vi "输入数据解析.vi"(0 "单个参数补充":dbl, 1 "从板号":dbl=1.0, 2 "主板二维码":string="BNET01", 3 "从板二维码":string="BNET01", 5 "主板引用":refnum<vi>, 7 "从板引用":refnum<vi>, 9 "主板选项":string="三级故障阀值", 11 "枚举":enum16{"主板", "从板"}(ring), 12 "快换":bool caption="快换写入") -> (4 "输出数组":dbl[][](array[numeric]), 6 "数组长度":dbl[](array[numeric]), 8 "循环次数":i32, 10 "命令":u32, 14 "名称":string[](array[string]), 15 "命令序号":u32[](array[numeric]))   [LabVIEW 2013] (continued)
                n2255 = Unbundle By Name(w5791) -> ("SOC过低"=w5790:dbl)
                n2256 = call "输入分辨率计算-EV05.vi"("1字节?"=FALSE, "数值"=w5790, "偏移量"=0.0, "分辨率"=0.1) -> ("低字节"=w5788:dbl, "高字节1"=w5789:dbl)  [unwired: 1 in, 5 out]
                n2257 = call "二进制解析-8.6.vi"("索引"=4, "数值"=w5789) -> ("低位子数组"=w5787:i32[])  [unwired: 3 out]
                n2258 = disable-structure shown="启用" {
                  disable-tunnel: w5788 -> [w5798 _]
                  disable-tunnel: [w5798 255 ("高字节1")] -> w5786
                  disable-tunnel: w5787 -> [w5797 _]
                  frame Disabled {
                    (unwired) i32[] [] ("低位子数组 4")
                  }
                  frame Enabled {
                  }
                }
                n2259 = Build Array(w5786, w5786) -> (w5794:i32[])
              }
              frame 14 {
                # "内阻过大"
                n2260 = disable-structure shown="启用" {
                  disable-tunnel: w5802 -> [w5807 _]
                  disable-tunnel: [w5803 255 ("高字节1")] -> w5800
                  frame Disabled {
                    n2261 = Unbundle By Name(w5807) -> ("内阻过大"=w5806:dbl)
                    n2262 = call "输入分辨率计算-EV05.vi"("1字节?"=TRUE, "数值"=w5806, "分辨率"=0.1) -> ("高字节1"=w5803:dbl)  [unwired: 2 in, 6 out]
                  }
                  frame Enabled {
                  }
                }
                n2263 = Build Array(w5800) -> (w5801:i32[])
              }
              frame 15 {
                # "极柱温度过高"
                n2264 = disable-structure shown="启用" {
                  disable-tunnel: w5811 -> [w5817 _]
                  disable-tunnel: [w5813 255 ("高字节1")] -> w5809
                  frame Disabled {
                    n2265 = Unbundle By Name(w5817) -> ("极柱温度过高"=w5816:dbl)
                    n2266 = call "输入分辨率计算-EV05.vi"("1字节?"=TRUE, "数值"=w5816, "偏移量"=-40.0, "分辨率"=1.0) -> ("高字节1"=w5813:dbl)  [unwired: 1 in, 6 out]
                  }
                  frame Enabled {
                  }
                }
                n2267 = Build Array(w5809) -> (w5810:i32[])
              }
              frame 16 {
                # "SOH过低"
                n2268 = disable-structure shown="启用" {
                  disable-tunnel: [w5834 w5842] -> w5821
                  disable-tunnel: w5820 -> [w5831 _]
                  disable-tunnel: [w5823 w5842] -> w5819
                  frame Disabled {
                    n2269 = Unbundle By Name(w5831) -> ("SOH过低"=w5830:dbl)
                    n2270 = call "输入分辨率计算-EV05.vi"("1字节?"=FALSE, "数值"=w5830, "偏移量"=0.0, "分辨率"=0.1) -> ("低字节"=w5832:dbl, "高字节1"=w5833:dbl)  [unwired: 1 in, 5 out]
                    n2271 = call "二进制解析-8.6.vi"("索引"=4, "数值"=w5833) -> ("低位子数组"=w5836:i32[])  [unwired: 3 out]
                    n2272 = call "二进制解析-8.6.vi"("索引"=4, "数值"=w5832) -> ("低位子数组"=w5825:i32[], "高位子数组"=w5835:i32[])  [unwired: 2 out]
                    n2273 = call "二进制解析-8.6.vi"("索引"=4, "数值"=0) -> ("低位子数组"=w5826:i32[])  [unwired: 3 out]
                    n2274 = Insert Into Array(array=w5836, new element=w5835) -> (w5829:i32[])  [unwired: 1 in]
                    n2275 = Insert Into Array(array=w5825, new element=w5826) -> (w5824:i32[])  [unwired: 1 in]
                    n2276 = call "数值二进制转十进制-8.6.vi"("子数组"=w5829) -> ("十进制数值"=w5834:i32)  [unwired: 4 out]
                    n2277 = call "数值二进制转十进制-8.6.vi"("子数组"=w5824) -> ("十进制数值"=w5823:i32)  [unwired: 4 out]
                  }
                  frame Enabled {
                    w5842 = 255 ("高字节1")
                  }
                }
                n2278 = Build Array(w5821, w5819) -> (w5822:i32[])
              }
            }
            n2279 = Insert Into Array(array=w5628, new element=w5629) -> (w5627:dbl[])  [unwired: 1 in]
          }
          n2280 = Build Array(w5624) -> (w5623:dbl[][])
          n2281 = Build Array("三级故障阀值") -> (w5614:string[])
        }
        frame "单体电压过高" {
          n2282 = Unbundle By Name(w5848) -> ("一级故障"=w5849:refnum<vi>)
          n2283 = property class="Clust (严格)"(reference=w5849) -> ("Value"=w5847:T4)  [unwired: 1 in, 2 out]
          n2284 = for {
            N: 17 -> [_]
            tunnel: w5847 -> [w5859]
            shift-right: [w5856] -> w5853
            shift-left: dbl[] [] -> [w5857]
            i -> [w5860]
            n2285 = case shown="13" w5860 {
              tunnel: w5859 -> [w5861 w5872 w5883 w5893 w5903 w5913 w5925 w5937 w5949 w5961 w5973 w5985 w5999 w6020 w6032 w6041 w6050]
              tunnel: [w5862 w5873 w5884 w5894 w5904 w5915 w5927 w5939 w5951 w5963 w5975 w5986 w6008 w6023 w6031 w6040 w6052] -> w5858
              frame 0, Default {
                # "总电压过高"
                n2286 = disable-structure shown="启用" {
                  disable-tunnel: [w5868 w5871] -> w5864
                  disable-tunnel: [w5867 w5871] -> w5863
                  disable-tunnel: w5861 -> [w5866 _]
                  frame Disabled {
                    n2287 = Unbundle By Name(w5866) -> ("总电压过高"=w5865:dbl)
                    n2288 = call "输入分辨率计算-EV05.vi"("1字节?"=FALSE, "数值"=w5865, "分辨率"=0.1) -> ("低字节"=w5868:dbl, "高字节1"=w5867:dbl)  [unwired: 2 in, 5 out]
                  }
                  frame Enabled {
                    w5871 = 255 ("高字节1")
                  }
                }
                n2289 = Build Array(w5863, w5864) -> (w5862:i32[])
              }
              frame 1 {
                # "总电压过低"
                n2290 = disable-structure shown="启用" {
                  disable-tunnel: [w5879 w5882] -> w5875
                  disable-tunnel: [w5878 w5882] -> w5874
                  disable-tunnel: w5872 -> [w5877 _]
                  frame Disabled {
                    n2291 = Unbundle By Name(w5877) -> ("总电压过低"=w5876:dbl)
                    n2292 = call "输入分辨率计算-EV05.vi"("1字节?"=FALSE, "数值"=w5876, "分辨率"=0.1) -> ("低字节"=w5879:dbl, "高字节1"=w5878:dbl)  [unwired: 2 in, 5 out]
                  }
                  frame Enabled {
                    w5882 = 255 ("高字节1")
                  }
                }
                n2293 = Build Array(w5874, w5875) -> (w5873:i32[])
              }
              frame 2 {
                # "温度过高"
                n2294 = disable-structure shown="启用" {
                  disable-tunnel: [w5889 255 ("高字节1")] -> w5885
                  disable-tunnel: w5883 -> [w5887 _]
                  frame Disabled {
                    n2295 = Unbundle By Name(w5887) -> ("温度过高"=w5886:dbl)
                    n2296 = call "输入分辨率计算-EV05.vi"("1字节?"=TRUE, "数值"=w5886, "偏移量"=-40.0, "分辨率"=1.0) -> ("高字节1"=w5889:dbl)  [unwired: 1 in, 6 out]
                  }
                  frame Enabled {
                  }
                }
                n2297 = Build Array(w5885) -> (w5884:i32[])
              }
              frame 3 {
                # "温度过低"
                n2298 = disable-structure shown="启用" {
                  disable-tunnel: [w5899 255 ("高字节1")] -> w5895
                  disable-tunnel: w5893 -> [w5897 _]
                  frame Disabled {
                    n2299 = Unbundle By Name(w5897) -> ("温度过低"=w5896:dbl)
                    n2300 = call "输入分辨率计算-EV05.vi"("1字节?"=TRUE, "数值"=w5896, "偏移量"=-40.0, "分辨率"=1.0) -> ("高字节1"=w5899:dbl)  [unwired: 1 in, 6 out]
                  }
                  frame Enabled {
                  }
                }
                n2301 = Build Array(w5895) -> (w5894:i32[])
              }
              frame 4 {
                # "整组温度不均衡"
                n2302 = disable-structure shown="启用" {
                  disable-tunnel: [w5909 255 ("高字节1")] -> w5905
                  disable-tunnel: w5903 -> [w5907 _]
                  frame Disabled {
                    n2303 = Unbundle By Name(w5907) -> ("整组温度不均衡"=w5906:dbl)
                    n2304 = call "输入分辨率计算-EV05.vi"("1字节?"=TRUE, "数值"=w5906, "偏移量"=0.0, "分辨率"=1.0) -> ("高字节1"=w5909:dbl)  [unwired: 1 in, 6 out]
                  }
                  frame Enabled {
                  }
                }
                n2305 = Build Array(w5905) -> (w5904:i32[])
              }
              frame 5 {
                # "单组电压不均衡"
                n2306 = disable-structure shown="启用" {
                  disable-tunnel: [w5921 w5924] -> w5916
                  disable-tunnel: [w5919 w5924] -> w5914
                  disable-tunnel: w5913 -> [w5918 _]
                  frame Disabled {
                    n2307 = Unbundle By Name(w5918) -> ("单组电压不均衡"=w5917:dbl)
                    n2308 = call "输入分辨率计算-EV05.vi"("1字节?"=FALSE, "数值"=w5917, "偏移量"=0.0, "分辨率"=0.001) -> ("低字节"=w5919:dbl, "高字节1"=w5921:dbl)  [unwired: 1 in, 5 out]
                  }
                  frame Enabled {
                    w5924 = 255 ("高字节1")
                  }
                }
                n2309 = Build Array(w5916, w5914) -> (w5915:i32[])
              }
              frame 6 {
                # "整组电压不均衡"
                n2310 = disable-structure shown="启用" {
                  disable-tunnel: [w5933 w5936] -> w5928
                  disable-tunnel: [w5931 w5936] -> w5926
                  disable-tunnel: w5925 -> [w5930 _]
                  frame Disabled {
                    n2311 = Unbundle By Name(w5930) -> ("整组电压不均衡"=w5929:dbl)
                    n2312 = call "输入分辨率计算-EV05.vi"("1字节?"=FALSE, "数值"=w5929, "偏移量"=0.0, "分辨率"=0.001) -> ("低字节"=w5931:dbl, "高字节1"=w5933:dbl)  [unwired: 1 in, 5 out]
                  }
                  frame Enabled {
                    w5936 = 255 ("高字节1")
                  }
                }
                n2313 = Build Array(w5928, w5926) -> (w5927:i32[])
              }
              frame 7 {
                # "单体电压过高"
                n2314 = disable-structure shown="启用" {
                  disable-tunnel: [w5945 w5948] -> w5940
                  disable-tunnel: [w5943 w5948] -> w5938
                  disable-tunnel: w5937 -> [w5942 _]
                  frame Enabled {
                    n2315 = Unbundle By Name(w5942) -> ("单体电压过高"=w5941:dbl)
                    n2316 = call "输入分辨率计算-EV05.vi"("1字节?"=FALSE, "数值"=w5941, "偏移量"=0.0, "分辨率"=0.001) -> ("低字节"=w5943:dbl, "高字节1"=w5945:dbl)  [unwired: 1 in, 5 out]
                  }
                  frame Disabled {
                    w5948 = 255 ("高字节1")
                  }
                }
                n2317 = Build Array(w5940, w5938) -> (w5939:dbl[])
              }
              frame 8 {
                # "单体电压过低"
                n2318 = disable-structure shown="启用" {
                  disable-tunnel: [w5957 w5960] -> w5952
                  disable-tunnel: [w5955 w5960] -> w5950
                  disable-tunnel: w5949 -> [w5954 _]
                  frame Disabled {
                    n2319 = Unbundle By Name(w5954) -> ("单体电压过低"=w5953:dbl)
                    n2320 = call "输入分辨率计算-EV05.vi"("1字节?"=FALSE, "数值"=w5953, "偏移量"=0.0, "分辨率"=0.001) -> ("低字节"=w5955:dbl, "高字节1"=w5957:dbl)  [unwired: 1 in, 5 out]
                  }
                  frame Enabled {
                    w5960 = 255 ("高字节1")
                  }
                }
                n2321 = Build Array(w5952, w5950) -> (w5951:i32[])
              }
              frame 9 {
                # "充电电流过高"
                n2322 = disable-structure shown="启用" {
                  disable-tunnel: [w5969 w5972] -> w5964
                  disable-tunnel: [w5967 w5972] -> w5962
                  disable-tunnel: w5961 -> [w5966 _]
                  frame Disabled {
                    n2323 = Unbundle By Name(w5966) -> ("充电电流过高"=w5965:dbl)
                    n2324 = call "输入分辨率计算-EV05.vi"("1字节?"=FALSE, "数值"=w5965, "偏移量"=-3000.0, "分辨率"=0.1) -> ("低字节"=w5967:dbl, "高字节1"=w5969:dbl)  [unwired: 1 in, 5 out]
                  }
                  frame Enabled {
                    w5972 = 255 ("高字节1")
                  }
                }
                n2325 = Build Array(w5964, w5962) -> (w5963:i32[])
              }
              frame 10 {
                # "放电电流过高"
                n2326 = disable-structure shown="启用" {
                  disable-tunnel: [w5981 w5984] -> w5976
                  disable-tunnel: [w5979 w5984] -> w5974
                  disable-tunnel: w5973 -> [w5978 _]
                  frame Disabled {
                    n2327 = Unbundle By Name(w5978) -> ("放电电流过高"=w5977:dbl)
                    n2328 = call "输入分辨率计算-EV05.vi"("1字节?"=FALSE, "数值"=w5977, "偏移量"=-3000.0, "分辨率"=0.1) -> ("低字节"=w5979:dbl, "高字节1"=w5981:dbl)  [unwired: 1 in, 5 out]
                  }
                  frame Enabled {
                    w5984 = 255 ("高字节1")
                  }
                }
                n2329 = Build Array(w5976, w5974) -> (w5975:i32[])
              }
              frame 11 {
                # "单组温度不均衡"
                n2330 = disable-structure shown="启用" {
                  disable-tunnel: [w5991 255 ("高字节1")] -> w5987
                  disable-tunnel: w5985 -> [w5989 _]
                  frame Disabled {
                    n2331 = Unbundle By Name(w5989) -> ("单组温度不均衡"=w5988:dbl)
                    n2332 = call "输入分辨率计算-EV05.vi"("1字节?"=TRUE, "数值"=w5988, "偏移量"=0.0, "分辨率"=1.0) -> ("高字节1"=w5991:dbl)  [unwired: 1 in, 6 out]
                  }
                  frame Enabled {
                  }
                }
                n2333 = Build Array(w5987) -> (w5986:i32[])
              }
              frame 12 {
                # "SOC过高"
                n2334 = Unbundle By Name(w5999) -> ("SOC过高"=w5998:dbl)
                n2335 = call "输入分辨率计算-EV05.vi"("1字节?"=FALSE, "数值"=w5998, "偏移量"=0.0, "分辨率"=0.1) -> ("低字节"=w6000:dbl, "高字节1"=w6001:dbl)  [unwired: 1 in, 5 out]
                n2336 = call "二进制解析-8.6.vi"("索引"=4, "数值"=w6001) -> ("低位子数组"=w6004:i32[])  [unwired: 3 out]
                n2337 = call "二进制解析-8.6.vi"("索引"=4, "数值"=w6000) -> ("低位子数组"=w5996:i32[], "高位子数组"=w6003:i32[])  [unwired: 2 out]
                n2338 = Insert Into Array(array=w6004, new element=w6003) -> (w6002:i32[])  [unwired: 1 in]
                n2339 = call "数值二进制转十进制-8.6.vi"("子数组"=w6002) -> ("十进制数值"=w5997:i32)  [unwired: 4 out]
                n2340 = disable-structure shown="启用" {
                  disable-tunnel: w5997 -> [w6012 _]
                  disable-tunnel: [w6012 255 ("高字节1")] -> w5995
                  disable-tunnel: [w6011 i32[] [] ("低位子数组 25")] -> _
                  disable-tunnel: w5996 -> [w6011 _]
                  frame Disabled {
                  }
                  frame Enabled {
                  }
                }
                n2341 = Build Array(w5995, w5995) -> (w6008:i32[])
              }
              frame 13 {
                # "SOC过低"
                n2342 = Unbundle By Name(w6020) -> ("SOC过低"=w6019:dbl)
                n2343 = call "输入分辨率计算-EV05.vi"("1字节?"=FALSE, "数值"=w6019, "偏移量"=0.0, "分辨率"=0.1) -> ("低字节"=w6017:dbl, "高字节1"=w6018:dbl)  [unwired: 1 in, 5 out]
                n2344 = call "二进制解析-8.6.vi"("索引"=4, "数值"=w6018) -> ("低位子数组"=w6016:i32[])  [unwired: 3 out]
                n2345 = disable-structure shown="启用" {
                  disable-tunnel: w6017 -> [w6027 _]
                  disable-tunnel: [w6027 255 ("高字节1")] -> w6015
                  disable-tunnel: w6016 -> [w6026 _]
                  disable-tunnel: [w6026 i32[] [] ("低位子数组")] -> _
                  frame Disabled {
                    (unwired) i32[] [] ("低位子数组 4")
                  }
                  frame Enabled {
                  }
                }
                n2346 = Build Array(w6015, w6015) -> (w6023:i32[])
              }
              frame 14 {
                # "内阻过大"
                n2347 = disable-structure shown="启用" {
                  disable-tunnel: w6032 -> [w6037 _]
                  disable-tunnel: [w6033 255 ("高字节1")] -> w6030
                  frame Disabled {
                    n2348 = Unbundle By Name(w6037) -> ("内阻过大"=w6036:dbl)
                    n2349 = call "输入分辨率计算-EV05.vi"("1字节?"=TRUE, "数值"=w6036, "分辨率"=0.1) -> ("高字节1"=w6033:dbl)  [unwired: 2 in, 6 out]
                  }
                  frame Enabled {
                  }
                }
                n2350 = Build Array(w6030) -> (w6031:i32[])
              }
              frame 15 {
                # "极柱温度过高"
                n2351 = disable-structure shown="启用" {
                  disable-tunnel: w6041 -> [w6047 _]
                  disable-tunnel: [w6043 255 ("高字节1")] -> w6039
                  frame Disabled {
                    n2352 = Unbundle By Name(w6047) -> ("极柱温度过高"=w6046:dbl)
                    n2353 = call "输入分辨率计算-EV05.vi"("1字节?"=TRUE, "数值"=w6046, "偏移量"=-40.0, "分辨率"=1.0) -> ("高字节1"=w6043:dbl)  [unwired: 1 in, 6 out]
                  }
                  frame Enabled {
                  }
                }
                n2354 = Build Array(w6039) -> (w6040:i32[])
              }
              frame 16 {
                # "SOH过低"
                n2355 = disable-structure shown="启用" {
                  disable-tunnel: [w6064 w6072] -> w6051
                  disable-tunnel: w6050 -> [w6061 _]
                  disable-tunnel: [w6053 w6072] -> w6049
                  frame Disabled {
                    n2356 = Unbundle By Name(w6061) -> ("SOH过低"=w6060:dbl)
                    n2357 = call "输入分辨率计算-EV05.vi"("1字节?"=FALSE, "数值"=w6060, "偏移量"=0.0, "分辨率"=0.1) -> ("低字节"=w6062:dbl, "高字节1"=w6063:dbl)  [unwired: 1 in, 5 out]
                    n2358 = call "二进制解析-8.6.vi"("索引"=4, "数值"=w6063) -> ("低位子数组"=w6066:i32[])  [unwired: 3 out]
                    n2359 = call "二进制解析-8.6.vi"("索引"=4, "数值"=w6062) -> ("低位子数组"=w6055:i32[], "高位子数组"=w6065:i32[])  [unwired: 2 out]
                    n2360 = call "二进制解析-8.6.vi"("索引"=4, "数值"=0) -> ("低位子数组"=w6056:i32[])  [unwired: 3 out]
                    n2361 = Insert Into Array(array=w6066, new element=w6065) -> (w6059:i32[])  [unwired: 1 in]
                    n2362 = Insert Into Array(array=w6055, new element=w6056) -> (w6054:i32[])  [unwired: 1 in]
                    n2363 = call "数值二进制转十进制-8.6.vi"("子数组"=w6059) -> ("十进制数值"=w6064:i32)  [unwired: 4 out]
                    n2364 = call "数值二进制转十进制-8.6.vi"("子数组"=w6054) -> ("十进制数值"=w6053:i32)  [unwired: 4 out]
                  }
                  frame Enabled {
                    w6072 = 255 ("高字节1")
                  }
                }
                n2365 = Build Array(w6051, w6049) -> (w6052:i32[])
              }
            }
            n2366 = Insert Into Array(array=w5857, new element=w5858) -> (w5856:dbl[])  [unwired: 1 in]
          }
          n2367 = Build Array(w5853) -> (w5852:dbl[][])
          n2368 = Build Array("一级故障阀值") -> (w5843:string[])
        }
        frame "单体电压过高(2)" {
          n2369 = Unbundle By Name(w6078) -> ("一级故障 2"=w6079:refnum<vi>)
          n2370 = property class="Clust (严格)"(reference=w6079) -> ("Value"=w6077:T4)  [unwired: 1 in, 2 out]
          n2371 = for {
            N: 17 -> [_]
            tunnel: w6077 -> [w6089]
            shift-right: [w6086] -> w6083
            shift-left: dbl[] [] -> [w6087]
            i -> [w6090]
            n2372 = case shown="13" w6090 {
              tunnel: w6089 -> [w6091 w6102 w6113 w6123 w6133 w6143 w6155 w6167 w6179 w6191 w6203 w6215 w6229 w6250 w6262 w6271 w6280]
              tunnel: [w6092 w6103 w6114 w6124 w6134 w6145 w6157 w6169 w6181 w6193 w6205 w6216 w6238 w6253 w6261 w6270 w6282] -> w6088
              frame 0, Default {
                # "总电压过高"
                n2373 = disable-structure shown="启用" {
                  disable-tunnel: [w6098 w6101] -> w6094
                  disable-tunnel: [w6097 w6101] -> w6093
                  disable-tunnel: w6091 -> [w6096 _]
                  frame Disabled {
                    n2374 = Unbundle By Name(w6096) -> ("总电压过高"=w6095:dbl)
                    n2375 = call "输入分辨率计算-EV05.vi"("1字节?"=FALSE, "数值"=w6095, "分辨率"=0.1) -> ("低字节"=w6098:dbl, "高字节1"=w6097:dbl)  [unwired: 2 in, 5 out]
                  }
                  frame Enabled {
                    w6101 = 255 ("高字节1")
                  }
                }
                n2376 = Build Array(w6093, w6094) -> (w6092:i32[])
              }
              frame 1 {
                # "总电压过低"
                n2377 = disable-structure shown="启用" {
                  disable-tunnel: [w6109 w6112] -> w6105
                  disable-tunnel: [w6108 w6112] -> w6104
                  disable-tunnel: w6102 -> [w6107 _]
                  frame Disabled {
                    n2378 = Unbundle By Name(w6107) -> ("总电压过低"=w6106:dbl)
                    n2379 = call "输入分辨率计算-EV05.vi"("1字节?"=FALSE, "数值"=w6106, "分辨率"=0.1) -> ("低字节"=w6109:dbl, "高字节1"=w6108:dbl)  [unwired: 2 in, 5 out]
                  }
                  frame Enabled {
                    w6112 = 255 ("高字节1")
                  }
                }
                n2380 = Build Array(w6104, w6105) -> (w6103:i32[])
              }
              frame 2 {
                # "温度过高"
                n2381 = disable-structure shown="启用" {
                  disable-tunnel: [w6119 255 ("高字节1")] -> w6115
                  disable-tunnel: w6113 -> [w6117 _]
                  frame Disabled {
                    n2382 = Unbundle By Name(w6117) -> ("温度过高"=w6116:dbl)
                    n2383 = call "输入分辨率计算-EV05.vi"("1字节?"=TRUE, "数值"=w6116, "偏移量"=-40.0, "分辨率"=1.0) -> ("高字节1"=w6119:dbl)  [unwired: 1 in, 6 out]
                  }
                  frame Enabled {
                  }
                }
                n2384 = Build Array(w6115) -> (w6114:i32[])
              }
              frame 3 {
                # "温度过低"
                n2385 = disable-structure shown="启用" {
                  disable-tunnel: [w6129 255 ("高字节1")] -> w6125
                  disable-tunnel: w6123 -> [w6127 _]
                  frame Disabled {
                    n2386 = Unbundle By Name(w6127) -> ("温度过低"=w6126:dbl)
                    n2387 = call "输入分辨率计算-EV05.vi"("1字节?"=TRUE, "数值"=w6126, "偏移量"=-40.0, "分辨率"=1.0) -> ("高字节1"=w6129:dbl)  [unwired: 1 in, 6 out]
                  }
                  frame Enabled {
                  }
                }
                n2388 = Build Array(w6125) -> (w6124:i32[])
              }
              frame 4 {
                # "整组温度不均衡"
                n2389 = disable-structure shown="启用" {
                  disable-tunnel: [w6139 255 ("高字节1")] -> w6135
                  disable-tunnel: w6133 -> [w6137 _]
                  frame Disabled {
                    n2390 = Unbundle By Name(w6137) -> ("整组温度不均衡"=w6136:dbl)
                    n2391 = call "输入分辨率计算-EV05.vi"("1字节?"=TRUE, "数值"=w6136, "偏移量"=0.0, "分辨率"=1.0) -> ("高字节1"=w6139:dbl)  [unwired: 1 in, 6 out]
                  }
                  frame Enabled {
                  }
                }
                n2392 = Build Array(w6135) -> (w6134:i32[])
              }
              frame 5 {
                # "单组电压不均衡"
                n2393 = disable-structure shown="启用" {
                  disable-tunnel: [w6151 w6154] -> w6146
                  disable-tunnel: [w6149 w6154] -> w6144
                  disable-tunnel: w6143 -> [w6148 _]
                  frame Disabled {
                    n2394 = Unbundle By Name(w6148) -> ("单组电压不均衡"=w6147:dbl)
                    n2395 = call "输入分辨率计算-EV05.vi"("1字节?"=FALSE, "数值"=w6147, "偏移量"=0.0, "分辨率"=0.001) -> ("低字节"=w6149:dbl, "高字节1"=w6151:dbl)  [unwired: 1 in, 5 out]
                  }
                  frame Enabled {
                    w6154 = 255 ("高字节1")
                  }
                }
                n2396 = Build Array(w6146, w6144) -> (w6145:i32[])
              }
              frame 6 {
                # "整组电压不均衡"
                n2397 = disable-structure shown="启用" {
                  disable-tunnel: [w6163 w6166] -> w6158
                  disable-tunnel: [w6161 w6166] -> w6156
                  disable-tunnel: w6155 -> [w6160 _]
                  frame Disabled {
                    n2398 = Unbundle By Name(w6160) -> ("整组电压不均衡"=w6159:dbl)
                    n2399 = call "输入分辨率计算-EV05.vi"("1字节?"=FALSE, "数值"=w6159, "偏移量"=0.0, "分辨率"=0.001) -> ("低字节"=w6161:dbl, "高字节1"=w6163:dbl)  [unwired: 1 in, 5 out]
                  }
                  frame Enabled {
                    w6166 = 255 ("高字节1")
                  }
                }
                n2400 = Build Array(w6158, w6156) -> (w6157:i32[])
              }
              frame 7 {
                # "单体电压过高"
                n2401 = disable-structure shown="启用" {
                  disable-tunnel: [w6175 w6178] -> w6170
                  disable-tunnel: [w6173 w6178] -> w6168
                  disable-tunnel: w6167 -> [w6172 _]
                  frame Enabled {
                    n2402 = Unbundle By Name(w6172) -> ("单体电压过高"=w6171:dbl)
                    n2403 = call "输入分辨率计算-EV05.vi"("1字节?"=FALSE, "数值"=w6171, "偏移量"=0.0, "分辨率"=0.001) -> ("低字节"=w6173:dbl, "高字节1"=w6175:dbl)  [unwired: 1 in, 5 out]
                  }
                  frame Disabled {
                    w6178 = 255 ("高字节1")
                  }
                }
                n2404 = Build Array(w6170, w6168) -> (w6169:dbl[])
              }
              frame 8 {
                # "单体电压过低"
                n2405 = disable-structure shown="启用" {
                  disable-tunnel: [w6187 w6190] -> w6182
                  disable-tunnel: [w6185 w6190] -> w6180
                  disable-tunnel: w6179 -> [w6184 _]
                  frame Disabled {
                    n2406 = Unbundle By Name(w6184) -> ("单体电压过低"=w6183:dbl)
                    n2407 = call "输入分辨率计算-EV05.vi"("1字节?"=FALSE, "数值"=w6183, "偏移量"=0.0, "分辨率"=0.001) -> ("低字节"=w6185:dbl, "高字节1"=w6187:dbl)  [unwired: 1 in, 5 out]
                  }
                  frame Enabled {
                    w6190 = 255 ("高字节1")
                  }
                }
                n2408 = Build Array(w6182, w6180) -> (w6181:i32[])
              }
              frame 9 {
                # "充电电流过高"
                n2409 = disable-structure shown="启用" {
                  disable-tunnel: [w6199 w6202] -> w6194
                  disable-tunnel: [w6197 w6202] -> w6192
                  disable-tunnel: w6191 -> [w6196 _]
                  frame Disabled {
                    n2410 = Unbundle By Name(w6196) -> ("充电电流过高"=w6195:dbl)
                    n2411 = call "输入分辨率计算-EV05.vi"("1字节?"=FALSE, "数值"=w6195, "偏移量"=-3000.0, "分辨率"=0.1) -> ("低字节"=w6197:dbl, "高字节1"=w6199:dbl)  [unwired: 1 in, 5 out]
                  }
                  frame Enabled {
                    w6202 = 255 ("高字节1")
                  }
                }
                n2412 = Build Array(w6194, w6192) -> (w6193:i32[])
              }
              frame 10 {
                # "放电电流过高"
                n2413 = disable-structure shown="启用" {
                  disable-tunnel: [w6211 w6214] -> w6206
                  disable-tunnel: [w6209 w6214] -> w6204
                  disable-tunnel: w6203 -> [w6208 _]
                  frame Disabled {
                    n2414 = Unbundle By Name(w6208) -> ("放电电流过高"=w6207:dbl)
                    n2415 = call "输入分辨率计算-EV05.vi"("1字节?"=FALSE, "数值"=w6207, "偏移量"=-3000.0, "分辨率"=0.1) -> ("低字节"=w6209:dbl, "高字节1"=w6211:dbl)  [unwired: 1 in, 5 out]
                  }
                  frame Enabled {
                    w6214 = 255 ("高字节1")
                  }
                }
                n2416 = Build Array(w6206, w6204) -> (w6205:i32[])
              }
              frame 11 {
                # "单组温度不均衡"
                n2417 = disable-structure shown="启用" {
                  disable-tunnel: [w6221 255 ("高字节1")] -> w6217
                  disable-tunnel: w6215 -> [w6219 _]
                  frame Disabled {
                    n2418 = Unbundle By Name(w6219) -> ("单组温度不均衡"=w6218:dbl)
                    n2419 = call "输入分辨率计算-EV05.vi"("1字节?"=TRUE, "数值"=w6218, "偏移量"=0.0, "分辨率"=1.0) -> ("高字节1"=w6221:dbl)  [unwired: 1 in, 6 out]
                  }
                  frame Enabled {
                  }
                }
                n2420 = Build Array(w6217) -> (w6216:i32[])
              }
              frame 12 {
                # "SOC过高"
                n2421 = Unbundle By Name(w6229) -> ("SOC过高"=w6228:dbl)
                n2422 = call "输入分辨率计算-EV05.vi"("1字节?"=FALSE, "数值"=w6228, "偏移量"=0.0, "分辨率"=0.1) -> ("低字节"=w6230:dbl, "高字节1"=w6231:dbl)  [unwired: 1 in, 5 out]
                n2423 = call "二进制解析-8.6.vi"("索引"=4, "数值"=w6231) -> ("低位子数组"=w6234:i32[])  [unwired: 3 out]
                n2424 = call "二进制解析-8.6.vi"("索引"=4, "数值"=w6230) -> ("低位子数组"=w6226:i32[], "高位子数组"=w6233:i32[])  [unwired: 2 out]
                n2425 = Insert Into Array(array=w6234, new element=w6233) -> (w6232:i32[])  [unwired: 1 in]
                n2426 = call "数值二进制转十进制-8.6.vi"("子数组"=w6232) -> ("十进制数值"=w6227:i32)  [unwired: 4 out]
                n2427 = disable-structure shown="启用" {
                  disable-tunnel: w6227 -> [w6242 _]
                  disable-tunnel: [w6242 255 ("高字节1")] -> w6225
                  disable-tunnel: [w6241 i32[] [] ("低位子数组 25")] -> _
                  disable-tunnel: w6226 -> [w6241 _]
                  frame Disabled {
                  }
                  frame Enabled {
                  }
                }
                n2428 = Build Array(w6225, w6225) -> (w6238:i32[])
              }
              frame 13 {
                # "SOC过低"
                n2429 = Unbundle By Name(w6250) -> ("SOC过低"=w6249:dbl)
                n2430 = call "输入分辨率计算-EV05.vi"("1字节?"=FALSE, "数值"=w6249, "偏移量"=0.0, "分辨率"=0.1) -> ("低字节"=w6247:dbl, "高字节1"=w6248:dbl)  [unwired: 1 in, 5 out]
                n2431 = call "二进制解析-8.6.vi"("索引"=4, "数值"=w6248) -> ("低位子数组"=w6246:i32[])  [unwired: 3 out]
                n2432 = disable-structure shown="启用" {
                  disable-tunnel: w6247 -> [w6257 _]
                  disable-tunnel: [w6257 255 ("高字节1")] -> w6245
                  disable-tunnel: w6246 -> [w6256 _]
                  disable-tunnel: [w6256 i32[] [] ("低位子数组")] -> _
                  frame Disabled {
                    (unwired) i32[] [] ("低位子数组 4")
                  }
                  frame Enabled {
                  }
                }
                n2433 = Build Array(w6245, w6245) -> (w6253:i32[])
              }
              frame 14 {
                # "内阻过大"
                n2434 = disable-structure shown="启用" {
                  disable-tunnel: w6262 -> [w6267 _]
                  disable-tunnel: [w6263 255 ("高字节1")] -> w6260
                  frame Disabled {
                    n2435 = Unbundle By Name(w6267) -> ("内阻过大"=w6266:dbl)
                    n2436 = call "输入分辨率计算-EV05.vi"("1字节?"=TRUE, "数值"=w6266, "分辨率"=0.1) -> ("高字节1"=w6263:dbl)  [unwired: 2 in, 6 out]
                  }
                  frame Enabled {
                  }
                }
                n2437 = Build Array(w6260) -> (w6261:i32[])
              }
              frame 15 {
                # "极柱温度过高"
                n2438 = disable-structure shown="启用" {
                  disable-tunnel: w6271 -> [w6277 _]
                  disable-tunnel: [w6273 255 ("高字节1")] -> w6269
                  frame Disabled {
                    n2439 = Unbundle By Name(w6277) -> ("极柱温度过高"=w6276:dbl)
                    n2440 = call "输入分辨率计算-EV05.vi"("1字节?"=TRUE, "数值"=w6276, "偏移量"=-40.0, "分辨率"=1.0) -> ("高字节1"=w6273:dbl)  [unwired: 1 in, 6 out]
                  }
                  frame Enabled {
                  }
                }
                n2441 = Build Array(w6269) -> (w6270:i32[])
              }
              frame 16 {
                # "SOH过低"
                n2442 = disable-structure shown="启用" {
                  disable-tunnel: [w6294 w6302] -> w6281
                  disable-tunnel: w6280 -> [w6291 _]
                  disable-tunnel: [w6283 w6302] -> w6279
                  frame Disabled {
                    n2443 = Unbundle By Name(w6291) -> ("SOH过低"=w6290:dbl)
                    n2444 = call "输入分辨率计算-EV05.vi"("1字节?"=FALSE, "数值"=w6290, "偏移量"=0.0, "分辨率"=0.1) -> ("低字节"=w6292:dbl, "高字节1"=w6293:dbl)  [unwired: 1 in, 5 out]
                    n2445 = call "二进制解析-8.6.vi"("索引"=4, "数值"=w6293) -> ("低位子数组"=w6296:i32[])  [unwired: 3 out]
                    n2446 = call "二进制解析-8.6.vi"("索引"=4, "数值"=w6292) -> ("低位子数组"=w6285:i32[], "高位子数组"=w6295:i32[])  [unwired: 2 out]
                    n2447 = call "二进制解析-8.6.vi"("索引"=4, "数值"=0) -> ("低位子数组"=w6286:i32[])  [unwired: 3 out]
                    n2448 = Insert Into Array(array=w6296, new element=w6295) -> (w6289:i32[])  [unwired: 1 in]
                    n2449 = Insert Into Array(array=w6285, new element=w6286) -> (w6284:i32[])  [unwired: 1 in]
                    n2450 = call "数值二进制转十进制-8.6.vi"("子数组"=w6289) -> ("十进制数值"=w6294:i32)  [unwired: 4 out]
                    n2451 = call "数值二进制转十进制-8.6.vi"("子数组"=w6284) -> ("十进制数值"=w6283:i32)  [unwired: 4 out]
                  }
                  frame Enabled {
                    w6302 = 255 ("高字节1")
                  }
                }
                n2452 = Build Array(w6281, w6279) -> (w6282:i32[])
              }
            }
            n2453 = Insert Into Array(array=w6087, new element=w6088) -> (w6086:dbl[])  [unwired: 1 in]
          }
          n2454 = Build Array(w6083) -> (w6082:dbl[][])
          n2455 = Build Array("二级故障阀值") -> (w6073:string[])
        }
        frame "单体电压过高(3)" {
          n2456 = Unbundle By Name(w6308) -> ("一级故障 3"=w6309:refnum<vi>)
          n2457 = property class="Clust (严格)"(reference=w6309) -> ("Value"=w6307:T4)  [unwired: 1 in, 2 out]
          n2458 = for {
            N: 17 -> [_]
            tunnel: w6307 -> [w6319]
            shift-right: [w6316] -> w6313
            shift-left: dbl[] [] -> [w6317]
            i -> [w6320]
            n2459 = case shown="13" w6320 {
              tunnel: w6319 -> [w6321 w6332 w6343 w6353 w6363 w6373 w6385 w6397 w6409 w6421 w6433 w6445 w6459 w6480 w6492 w6501 w6510]
              tunnel: [w6322 w6333 w6344 w6354 w6364 w6375 w6387 w6399 w6411 w6423 w6435 w6446 w6468 w6483 w6491 w6500 w6512] -> w6318
              frame 0, Default {
                # "总电压过高"
                n2460 = disable-structure shown="启用" {
                  disable-tunnel: [w6328 w6331] -> w6324
                  disable-tunnel: [w6327 w6331] -> w6323
                  disable-tunnel: w6321 -> [w6326 _]
                  frame Disabled {
                    n2461 = Unbundle By Name(w6326) -> ("总电压过高"=w6325:dbl)
                    n2462 = call "输入分辨率计算-EV05.vi"("1字节?"=FALSE, "数值"=w6325, "分辨率"=0.1) -> ("低字节"=w6328:dbl, "高字节1"=w6327:dbl)  [unwired: 2 in, 5 out]
                  }
                  frame Enabled {
                    w6331 = 255 ("高字节1")
                  }
                }
                n2463 = Build Array(w6323, w6324) -> (w6322:i32[])
              }
              frame 1 {
                # "总电压过低"
                n2464 = disable-structure shown="启用" {
                  disable-tunnel: [w6339 w6342] -> w6335
                  disable-tunnel: [w6338 w6342] -> w6334
                  disable-tunnel: w6332 -> [w6337 _]
                  frame Disabled {
                    n2465 = Unbundle By Name(w6337) -> ("总电压过低"=w6336:dbl)
                    n2466 = call "输入分辨率计算-EV05.vi"("1字节?"=FALSE, "数值"=w6336, "分辨率"=0.1) -> ("低字节"=w6339:dbl, "高字节1"=w6338:dbl)  [unwired: 2 in, 5 out]
                  }
                  frame Enabled {
                    w6342 = 255 ("高字节1")
                  }
                }
                n2467 = Build Array(w6334, w6335) -> (w6333:i32[])
              }
              frame 2 {
                # "温度过高"
                n2468 = disable-structure shown="启用" {
                  disable-tunnel: [w6349 255 ("高字节1")] -> w6345
                  disable-tunnel: w6343 -> [w6347 _]
                  frame Disabled {
                    n2469 = Unbundle By Name(w6347) -> ("温度过高"=w6346:dbl)
                    n2470 = call "输入分辨率计算-EV05.vi"("1字节?"=TRUE, "数值"=w6346, "偏移量"=-40.0, "分辨率"=1.0) -> ("高字节1"=w6349:dbl)  [unwired: 1 in, 6 out]
                  }
                  frame Enabled {
                  }
                }
                n2471 = Build Array(w6345) -> (w6344:i32[])
              }
              frame 3 {
                # "温度过低"
                n2472 = disable-structure shown="启用" {
                  disable-tunnel: [w6359 255 ("高字节1")] -> w6355
                  disable-tunnel: w6353 -> [w6357 _]
                  frame Disabled {
                    n2473 = Unbundle By Name(w6357) -> ("温度过低"=w6356:dbl)
                    n2474 = call "输入分辨率计算-EV05.vi"("1字节?"=TRUE, "数值"=w6356, "偏移量"=-40.0, "分辨率"=1.0) -> ("高字节1"=w6359:dbl)  [unwired: 1 in, 6 out]
                  }
                  frame Enabled {
                  }
                }
                n2475 = Build Array(w6355) -> (w6354:i32[])
              }
              frame 4 {
                # "整组温度不均衡"
                n2476 = disable-structure shown="启用" {
                  disable-tunnel: [w6369 255 ("高字节1")] -> w6365
                  disable-tunnel: w6363 -> [w6367 _]
                  frame Disabled {
                    n2477 = Unbundle By Name(w6367) -> ("整组温度不均衡"=w6366:dbl)
                    n2478 = call "输入分辨率计算-EV05.vi"("1字节?"=TRUE, "数值"=w6366, "偏移量"=0.0, "分辨率"=1.0) -> ("高字节1"=w6369:dbl)  [unwired: 1 in, 6 out]
                  }
                  frame Enabled {
                  }
                }
                n2479 = Build Array(w6365) -> (w6364:i32[])
              }
              frame 5 {
                # "单组电压不均衡"
                n2480 = disable-structure shown="启用" {
                  disable-tunnel: [w6381 w6384] -> w6376
                  disable-tunnel: [w6379 w6384] -> w6374
                  disable-tunnel: w6373 -> [w6378 _]
                  frame Disabled {
                    n2481 = Unbundle By Name(w6378) -> ("单组电压不均衡"=w6377:dbl)
                    n2482 = call "输入分辨率计算-EV05.vi"("1字节?"=FALSE, "数值"=w6377, "偏移量"=0.0, "分辨率"=0.001) -> ("低字节"=w6379:dbl, "高字节1"=w6381:dbl)  [unwired: 1 in, 5 out]
                  }
                  frame Enabled {
                    w6384 = 255 ("高字节1")
                  }
                }
                n2483 = Build Array(w6376, w6374) -> (w6375:i32[])
              }
              frame 6 {
                # "整组电压不均衡"
                n2484 = disable-structure shown="启用" {
                  disable-tunnel: [w6393 w6396] -> w6388
                  disable-tunnel: [w6391 w6396] -> w6386
                  disable-tunnel: w6385 -> [w6390 _]
                  frame Disabled {
                    n2485 = Unbundle By Name(w6390) -> ("整组电压不均衡"=w6389:dbl)
                    n2486 = call "输入分辨率计算-EV05.vi"("1字节?"=FALSE, "数值"=w6389, "偏移量"=0.0, "分辨率"=0.001) -> ("低字节"=w6391:dbl, "高字节1"=w6393:dbl)  [unwired: 1 in, 5 out]
                  }
                  frame Enabled {
                    w6396 = 255 ("高字节1")
                  }
                }
                n2487 = Build Array(w6388, w6386) -> (w6387:i32[])
              }
              frame 7 {
                # "单体电压过高"
                n2488 = disable-structure shown="启用" {
                  disable-tunnel: [w6405 w6408] -> w6400
                  disable-tunnel: [w6403 w6408] -> w6398
                  disable-tunnel: w6397 -> [w6402 _]
                  frame Enabled {
                    n2489 = Unbundle By Name(w6402) -> ("单体电压过高"=w6401:dbl)
                    n2490 = call "输入分辨率计算-EV05.vi"("1字节?"=FALSE, "数值"=w6401, "偏移量"=0.0, "分辨率"=0.001) -> ("低字节"=w6403:dbl, "高字节1"=w6405:dbl)  [unwired: 1 in, 5 out]
                  }
                  frame Disabled {
                    w6408 = 255 ("高字节1")
                  }
                }
                n2491 = Build Array(w6400, w6398) -> (w6399:dbl[])
              }
              frame 8 {
                # "单体电压过低"
                n2492 = disable-structure shown="启用" {
                  disable-tunnel: [w6417 w6420] -> w6412
                  disable-tunnel: [w6415 w6420] -> w6410
                  disable-tunnel: w6409 -> [w6414 _]
                  frame Disabled {
                    n2493 = Unbundle By Name(w6414) -> ("单体电压过低"=w6413:dbl)
                    n2494 = call "输入分辨率计算-EV05.vi"("1字节?"=FALSE, "数值"=w6413, "偏移量"=0.0, "分辨率"=0.001) -> ("低字节"=w6415:dbl, "高字节1"=w6417:dbl)  [unwired: 1 in, 5 out]
                  }
                  frame Enabled {
                    w6420 = 255 ("高字节1")
                  }
                }
                n2495 = Build Array(w6412, w6410) -> (w6411:i32[])
              }
              frame 9 {
                # "充电电流过高"
                n2496 = disable-structure shown="启用" {
                  disable-tunnel: [w6429 w6432] -> w6424
                  disable-tunnel: [w6427 w6432] -> w6422
                  disable-tunnel: w6421 -> [w6426 _]
                  frame Disabled {
                    n2497 = Unbundle By Name(w6426) -> ("充电电流过高"=w6425:dbl)
                    n2498 = call "输入分辨率计算-EV05.vi"("1字节?"=FALSE, "数值"=w6425, "偏移量"=-3000.0, "分辨率"=0.1) -> ("低字节"=w6427:dbl, "高字节1"=w6429:dbl)  [unwired: 1 in, 5 out]
                  }
                  frame Enabled {
                    w6432 = 255 ("高字节1")
                  }
                }
                n2499 = Build Array(w6424, w6422) -> (w6423:i32[])
              }
              frame 10 {
                # "放电电流过高"
                n2500 = disable-structure shown="启用" {
                  disable-tunnel: [w6441 w6444] -> w6436
                  disable-tunnel: [w6439 w6444] -> w6434
                  disable-tunnel: w6433 -> [w6438 _]
                  frame Disabled {
                    n2501 = Unbundle By Name(w6438) -> ("放电电流过高"=w6437:dbl)
                    n2502 = call "输入分辨率计算-EV05.vi"("1字节?"=FALSE, "数值"=w6437, "偏移量"=-3000.0, "分辨率"=0.1) -> ("低字节"=w6439:dbl, "高字节1"=w6441:dbl)  [unwired: 1 in, 5 out]
                  }
                  frame Enabled {
                    w6444 = 255 ("高字节1")
                  }
                }
                n2503 = Build Array(w6436, w6434) -> (w6435:i32[])
              }
              frame 11 {
                # "单组温度不均衡"
                n2504 = disable-structure shown="启用" {
                  disable-tunnel: [w6451 255 ("高字节1")] -> w6447
                  disable-tunnel: w6445 -> [w6449 _]
                  frame Disabled {
                    n2505 = Unbundle By Name(w6449) -> ("单组温度不均衡"=w6448:dbl)
                    n2506 = call "输入分辨率计算-EV05.vi"("1字节?"=TRUE, "数值"=w6448, "偏移量"=0.0, "分辨率"=1.0) -> ("高字节1"=w6451:dbl)  [unwired: 1 in, 6 out]
                  }
                  frame Enabled {
                  }
                }
                n2507 = Build Array(w6447) -> (w6446:i32[])
              }
              frame 12 {
                # "SOC过高"
                n2508 = Unbundle By Name(w6459) -> ("SOC过高"=w6458:dbl)
                n2509 = call "输入分辨率计算-EV05.vi"("1字节?"=FALSE, "数值"=w6458, "偏移量"=0.0, "分辨率"=0.1) -> ("低字节"=w6460:dbl, "高字节1"=w6461:dbl)  [unwired: 1 in, 5 out]
                n2510 = call "二进制解析-8.6.vi"("索引"=4, "数值"=w6461) -> ("低位子数组"=w6464:i32[])  [unwired: 3 out]
                n2511 = call "二进制解析-8.6.vi"("索引"=4, "数值"=w6460) -> ("低位子数组"=w6456:i32[], "高位子数组"=w6463:i32[])  [unwired: 2 out]
                n2512 = Insert Into Array(array=w6464, new element=w6463) -> (w6462:i32[])  [unwired: 1 in]
                n2513 = call "数值二进制转十进制-8.6.vi"("子数组"=w6462) -> ("十进制数值"=w6457:i32)  [unwired: 4 out]
                n2514 = disable-structure shown="启用" {
                  disable-tunnel: w6457 -> [w6472 _]
                  disable-tunnel: [w6472 255 ("高字节1")] -> w6455
                  disable-tunnel: [w6471 i32[] [] ("低位子数组 25")] -> _
                  disable-tunnel: w6456 -> [w6471 _]
                  frame Disabled {
                  }
                  frame Enabled {
                  }
                }
                n2515 = Build Array(w6455, w6455) -> (w6468:i32[])
              }
              frame 13 {
                # "SOC过低"
                n2516 = Unbundle By Name(w6480) -> ("SOC过低"=w6479:dbl)
                n2517 = call "输入分辨率计算-EV05.vi"("1字节?"=FALSE, "数值"=w6479, "偏移量"=0.0, "分辨率"=0.1) -> ("低字节"=w6477:dbl, "高字节1"=w6478:dbl)  [unwired: 1 in, 5 out]
                n2518 = call "二进制解析-8.6.vi"("索引"=4, "数值"=w6478) -> ("低位子数组"=w6476:i32[])  [unwired: 3 out]
                n2519 = disable-structure shown="启用" {
                  disable-tunnel: w6477 -> [w6487 _]
                  disable-tunnel: [w6487 255 ("高字节1")] -> w6475
                  disable-tunnel: w6476 -> [w6486 _]
                  disable-tunnel: [w6486 i32[] [] ("低位子数组")] -> _
                  frame Disabled {
                    (unwired) i32[] [] ("低位子数组 4")
                  }
                  frame Enabled {
                  }
                }
                n2520 = Build Array(w6475, w6475) -> (w6483:i32[])
              }
              frame 14 {
                # "内阻过大"
                n2521 = disable-structure shown="启用" {
                  disable-tunnel: w6492 -> [w6497 _]
                  disable-tunnel: [w6493 255 ("高字节1")] -> w6490
                  frame Disabled {
                    n2522 = Unbundle By Name(w6497) -> ("内阻过大"=w6496:dbl)
                    n2523 = call "输入分辨率计算-EV05.vi"("1字节?"=TRUE, "数值"=w6496, "分辨率"=0.1) -> ("高字节1"=w6493:dbl)  [unwired: 2 in, 6 out]
                  }
                  frame Enabled {
                  }
                }
                n2524 = Build Array(w6490) -> (w6491:i32[])
              }
              frame 15 {
                # "极柱温度过高"
                n2525 = disable-structure shown="启用" {
                  disable-tunnel: w6501 -> [w6507 _]
                  disable-tunnel: [w6503 255 ("高字节1")] -> w6499
                  frame Disabled {
                    n2526 = Unbundle By Name(w6507) -> ("极柱温度过高"=w6506:dbl)
                    n2527 = call "输入分辨率计算-EV05.vi"("1字节?"=TRUE, "数值"=w6506, "偏移量"=-40.0, "分辨率"=1.0) -> ("高字节1"=w6503:dbl)  [unwired: 1 in, 6 out]
                  }
                  frame Enabled {
                  }
                }
                n2528 = Build Array(w6499) -> (w6500:i32[])
              }
              frame 16 {
                # "SOH过低"
                n2529 = disable-structure shown="启用" {
                  disable-tunnel: [w6524 w6532] -> w6511
                  disable-tunnel: w6510 -> [w6521 _]
                  disable-tunnel: [w6513 w6532] -> w6509
                  frame Disabled {
                    n2530 = Unbundle By Name(w6521) -> ("SOH过低"=w6520:dbl)
                    n2531 = call "输入分辨率计算-EV05.vi"("1字节?"=FALSE, "数值"=w6520, "偏移量"=0.0, "分辨率"=0.1) -> ("低字节"=w6522:dbl, "高字节1"=w6523:dbl)  [unwired: 1 in, 5 out]
                    n2532 = call "二进制解析-8.6.vi"("索引"=4, "数值"=w6523) -> ("低位子数组"=w6526:i32[])  [unwired: 3 out]
                    n2533 = call "二进制解析-8.6.vi"("索引"=4, "数值"=w6522) -> ("低位子数组"=w6515:i32[], "高位子数组"=w6525:i32[])  [unwired: 2 out]
                    n2534 = call "二进制解析-8.6.vi"("索引"=4, "数值"=0) -> ("低位子数组"=w6516:i32[])  [unwired: 3 out]
                    n2535 = Insert Into Array(array=w6526, new element=w6525) -> (w6519:i32[])  [unwired: 1 in]
                    n2536 = Insert Into Array(array=w6515, new element=w6516) -> (w6514:i32[])  [unwired: 1 in]
                    n2537 = call "数值二进制转十进制-8.6.vi"("子数组"=w6519) -> ("十进制数值"=w6524:i32)  [unwired: 4 out]
                    n2538 = call "数值二进制转十进制-8.6.vi"("子数组"=w6514) -> ("十进制数值"=w6513:i32)  [unwired: 4 out]
                  }
                  frame Enabled {
                    w6532 = 255 ("高字节1")
                  }
                }
                n2539 = Build Array(w6511, w6509) -> (w6512:i32[])
              }
            }
            n2540 = Insert Into Array(array=w6317, new element=w6318) -> (w6316:dbl[])  [unwired: 1 in]
          }
          n2541 = Build Array(w6313) -> (w6312:dbl[][])
          n2542 = Build Array("三级故障阀值") -> (w6303:string[])
        }
        frame "单体电压过低" {
          n2543 = Unbundle By Name(w6538) -> ("一级故障"=w6539:refnum<vi>)
          n2544 = property class="Clust (严格)"(reference=w6539) -> ("Value"=w6537:T4)  [unwired: 1 in, 2 out]
          n2545 = for {
            N: 17 -> [_]
            tunnel: w6537 -> [w6549]
            shift-right: [w6546] -> w6543
            shift-left: dbl[] [] -> [w6547]
            i -> [w6550]
            n2546 = case shown="13" w6550 {
              tunnel: w6549 -> [w6551 w6562 w6573 w6583 w6593 w6603 w6615 w6627 w6639 w6651 w6663 w6675 w6689 w6710 w6721 w6730 w6739]
              tunnel: [w6552 w6563 w6574 w6584 w6594 w6605 w6617 w6629 w6641 w6653 w6665 w6676 w6698 w6713 w6720 w6729 w6741] -> w6548
              frame 0, Default {
                # "总电压过高"
                n2547 = disable-structure shown="启用" {
                  disable-tunnel: [w6558 w6561] -> w6554
                  disable-tunnel: [w6557 w6561] -> w6553
                  disable-tunnel: w6551 -> [w6556 _]
                  frame Disabled {
                    n2548 = Unbundle By Name(w6556) -> ("总电压过高"=w6555:dbl)
                    n2549 = call "输入分辨率计算-EV05.vi"("1字节?"=FALSE, "数值"=w6555, "分辨率"=0.1) -> ("低字节"=w6558:dbl, "高字节1"=w6557:dbl)  [unwired: 2 in, 5 out]
                  }
                  frame Enabled {
                    w6561 = 255 ("高字节1")
                  }
                }
                n2550 = Build Array(w6553, w6554) -> (w6552:i32[])
              }
              frame 1 {
                # "总电压过低"
                n2551 = disable-structure shown="启用" {
                  disable-tunnel: [w6569 w6572] -> w6565
                  disable-tunnel: [w6568 w6572] -> w6564
                  disable-tunnel: w6562 -> [w6567 _]
                  frame Disabled {
                    n2552 = Unbundle By Name(w6567) -> ("总电压过低"=w6566:dbl)
                    n2553 = call "输入分辨率计算-EV05.vi"("1字节?"=FALSE, "数值"=w6566, "分辨率"=0.1) -> ("低字节"=w6569:dbl, "高字节1"=w6568:dbl)  [unwired: 2 in, 5 out]
                  }
                  frame Enabled {
                    w6572 = 255 ("高字节1")
                  }
                }
                n2554 = Build Array(w6564, w6565) -> (w6563:i32[])
              }
              frame 2 {
                # "温度过高"
                n2555 = disable-structure shown="启用" {
                  disable-tunnel: [w6579 255 ("高字节1")] -> w6575
                  disable-tunnel: w6573 -> [w6577 _]
                  frame Disabled {
                    n2556 = Unbundle By Name(w6577) -> ("温度过高"=w6576:dbl)
                    n2557 = call "输入分辨率计算-EV05.vi"("1字节?"=TRUE, "数值"=w6576, "偏移量"=-40.0, "分辨率"=1.0) -> ("高字节1"=w6579:dbl)  [unwired: 1 in, 6 out]
                  }
                  frame Enabled {
                  }
                }
                n2558 = Build Array(w6575) -> (w6574:i32[])
              }
              frame 3 {
                # "温度过低"
                n2559 = disable-structure shown="启用" {
                  disable-tunnel: [w6589 255 ("高字节1")] -> w6585
                  disable-tunnel: w6583 -> [w6587 _]
                  frame Disabled {
                    n2560 = Unbundle By Name(w6587) -> ("温度过低"=w6586:dbl)
                    n2561 = call "输入分辨率计算-EV05.vi"("1字节?"=TRUE, "数值"=w6586, "偏移量"=-40.0, "分辨率"=1.0) -> ("高字节1"=w6589:dbl)  [unwired: 1 in, 6 out]
                  }
                  frame Enabled {
                  }
                }
                n2562 = Build Array(w6585) -> (w6584:i32[])
              }
              frame 4 {
                # "整组温度不均衡"
                n2563 = disable-structure shown="启用" {
                  disable-tunnel: [w6599 255 ("高字节1")] -> w6595
                  disable-tunnel: w6593 -> [w6597 _]
                  frame Disabled {
                    n2564 = Unbundle By Name(w6597) -> ("整组温度不均衡"=w6596:dbl)
                    n2565 = call "输入分辨率计算-EV05.vi"("1字节?"=TRUE, "数值"=w6596, "偏移量"=0.0, "分辨率"=1.0) -> ("高字节1"=w6599:dbl)  [unwired: 1 in, 6 out]
                  }
                  frame Enabled {
                  }
                }
                n2566 = Build Array(w6595) -> (w6594:i32[])
              }
              frame 5 {
                # "单组电压不均衡"
                n2567 = disable-structure shown="启用" {
                  disable-tunnel: [w6611 w6614] -> w6606
                  disable-tunnel: [w6609 w6614] -> w6604
                  disable-tunnel: w6603 -> [w6608 _]
                  frame Disabled {
                    n2568 = Unbundle By Name(w6608) -> ("单组电压不均衡"=w6607:dbl)
                    n2569 = call "输入分辨率计算-EV05.vi"("1字节?"=FALSE, "数值"=w6607, "偏移量"=0.0, "分辨率"=0.001) -> ("低字节"=w6609:dbl, "高字节1"=w6611:dbl)  [unwired: 1 in, 5 out]
                  }
                  frame Enabled {
                    w6614 = 255 ("高字节1")
                  }
                }
                n2570 = Build Array(w6606, w6604) -> (w6605:i32[])
              }
              frame 6 {
                # "整组电压不均衡"
                n2571 = disable-structure shown="启用" {
                  disable-tunnel: [w6623 w6626] -> w6618
